vi "get_calibration.vi"(8 "error in (no error)":errorcluster, 11 "ImageAssemblerDL090211Scaffold in":refnum<class "ImageAssemblerDL090211Scaffold.lvclass">) -> (0 "error out":errorcluster, 1 "y":dbl, 2 "x":dbl, 3 "ImageAssemblerDL090211Scaffold out":refnum<class "ImageAssemblerDL090211Scaffold.lvclass">, 5 "y unit":T1, 7 "x unit":T1)   [LabVIEW 2010, in "ImageAssemblerDL090211Scaffold.lvclass"]
uses:
  ImageAssemblerDL090211Scaffold.lvclass
  common/enumerations/unit.ctl
  ImageAssemblerDL090211Scaffold.lvclass/ImageAssemblerDL090211Scaffold.ctl
  common/classes/Image/Image/Image.lvclass
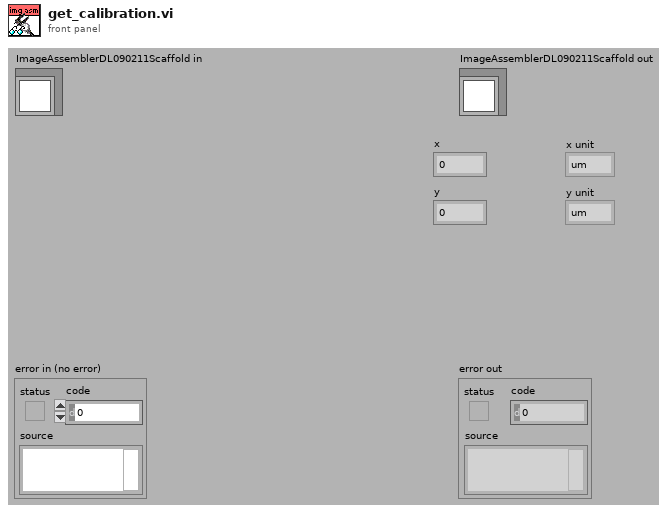
[diagram p1: front panel]
types:
  T1 = typedef "Image.lvclass/unit.ctl" = enum16{"um", "s"}
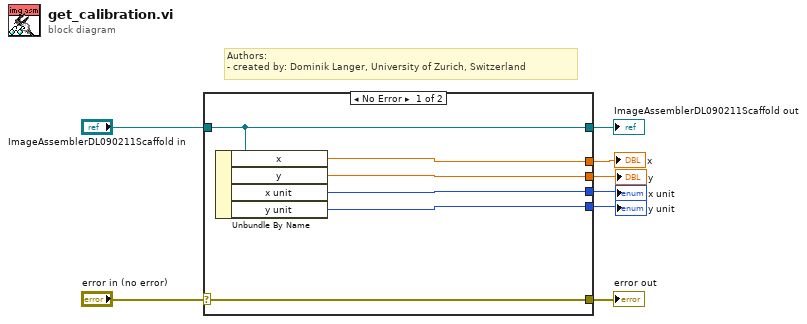
[diagram p0: block diagram]
diagram:
  # "Authors: \n- created by: Dominik Langer, University of Zurich, Switzerland"
  n1 = case shown="No Error" "error in (no error)" {
    selector: "error in (no error)" -> [w14 w15]
    tunnel: [w14 w15] -> w7
    tunnel: [w13 w16] -> w5
    tunnel: "ImageAssemblerDL090211Scaffold in" -> [w13 w16]
    tunnel: [w12 _] -> w4
    tunnel: [w11 _] -> w3
    tunnel: [w10 _] -> w2
    tunnel: [w9 _] -> w1
    frame No Error {
      n2 = Unbundle By Name(w13) -> ("x"=w12:dbl, "y"=w11:dbl, "x unit"=w10:T1, "y unit"=w9:T1)
    }
    frame Error {
    }
  }
  "error out" <- w7
  "ImageAssemblerDL090211Scaffold out" <- w5
  "y" <- w3
  "x" <- w4
  "x unit" <- w2
  "y unit" <- w1
